vi "Voltage - MeasureAF.vi"() -> ()   [LabVIEW 2017]
doc: "This example demonstrates how to continuously acquire buffered voltage measurements using a DAQmx device.\n\nFor instructions on how to connect your signals to the DAQ device, refer to your device documentation."
uses:
  <vilib>/Utility/error.llb/DialogType.ctl
  <vilib>/DAQmx/read.llb/DAQmx Read (Analog 1D Wfm NChan NSamp).vi
  <vilib>/DAQmx/write.llb/DAQmx Write (Analog 1D Wfm NChan NSamp).vi
  <vilib>/DAQmx/create/channels.llb/DAQmx Create Channel (AO-Voltage-Basic).vi
  <vilib>/DAQmx/configure/timing.llb/DAQmx Timing (Sample Clock).vi
  <vilib>/DAQmx/miscellaneous.llb/DAQmx Fill In Error Info.vi
  <vilib>/DAQmx/create/channels.llb/DAQmx Create Channel (AI-Voltage-Basic).vi
  <vilib>/DAQmx/configure/task.llb/DAQmx Configure Logging (TDMS).vi
  <vilib>/measure/matone.llb/Harmonic Distortion Analyzer N Chan.vi
  <vilib>/measure/matone.llb/Extract Single Tone Information N Chan.vi
  <vilib>/Utility/config.llb/Read Key (Double).vi
  <resource>/objmgr/daqmx.rc
  <vilib>/measure/NI_MAPro.lvlib
  <vilib>/Utility/config.llb/NI_LVConfig.lvlib
  <vilib>/measure/NI_MABase.lvlib
panel:
  out "c7":dbl
  out "c6":dbl
  out "c5":dbl
  out "c4":dbl
  out "c3":dbl
  out "c2":dbl
  out "c1":dbl
  out "c0":dbl
  out "Amplitudes":dbl[](array[numeric]) format="%.2p"
  out "Frequency":dbl[](array[numeric]) format="%.2p"
  out "Channel 7":waveform(dbl)(graph)
  out "Channel 6":waveform(dbl)(graph)
  out "Channel 5":waveform(dbl)(graph)
  out "Channel 4":waveform(dbl)(graph)
  out "Channel 3":waveform(dbl)(graph)
  out "Channel 2":waveform(dbl)(graph)
  out "Channel 1":waveform(dbl)(graph)
  out "Channel 0":waveform(dbl)(graph)
  out "FreqOut":dbl
  out "AmpOut":dbl
  in  "s":bool
  out "x = y?":bool
  in  "Number of Samples display":i32=1000
  in  "Stop 2":bool
  out "Actual Sample Rate 2":dbl=1000.0 format="%0.2f"
  out "Waveform Graph 3":waveform(dbl)[](graph)=[{"t0"=timestamp(0 s since 1904-01-01), "dt"=0.001, "Y"=[]}]
  out "THD":dbl[](array[numeric]) format="%.2p"
  out "Number Sample for avarage AF":i32
  out "stopAI":bool
  out "Time Stop App (s)":i32
  in  "Stop":bool
  out "Waveform Graph":waveform(dbl)[](graph)
  out "Actual Sample Rate":dbl=1000.0 format="%0.2f"
  # "Acquired Data"
  # "Channel0"
  # "Channel1"
  # "Channel2"
  # "Channel3"
  # "Channel4"
  # "Channel5"
  # "Channel6"
  # "Channel7"
  # "Timing Settings"
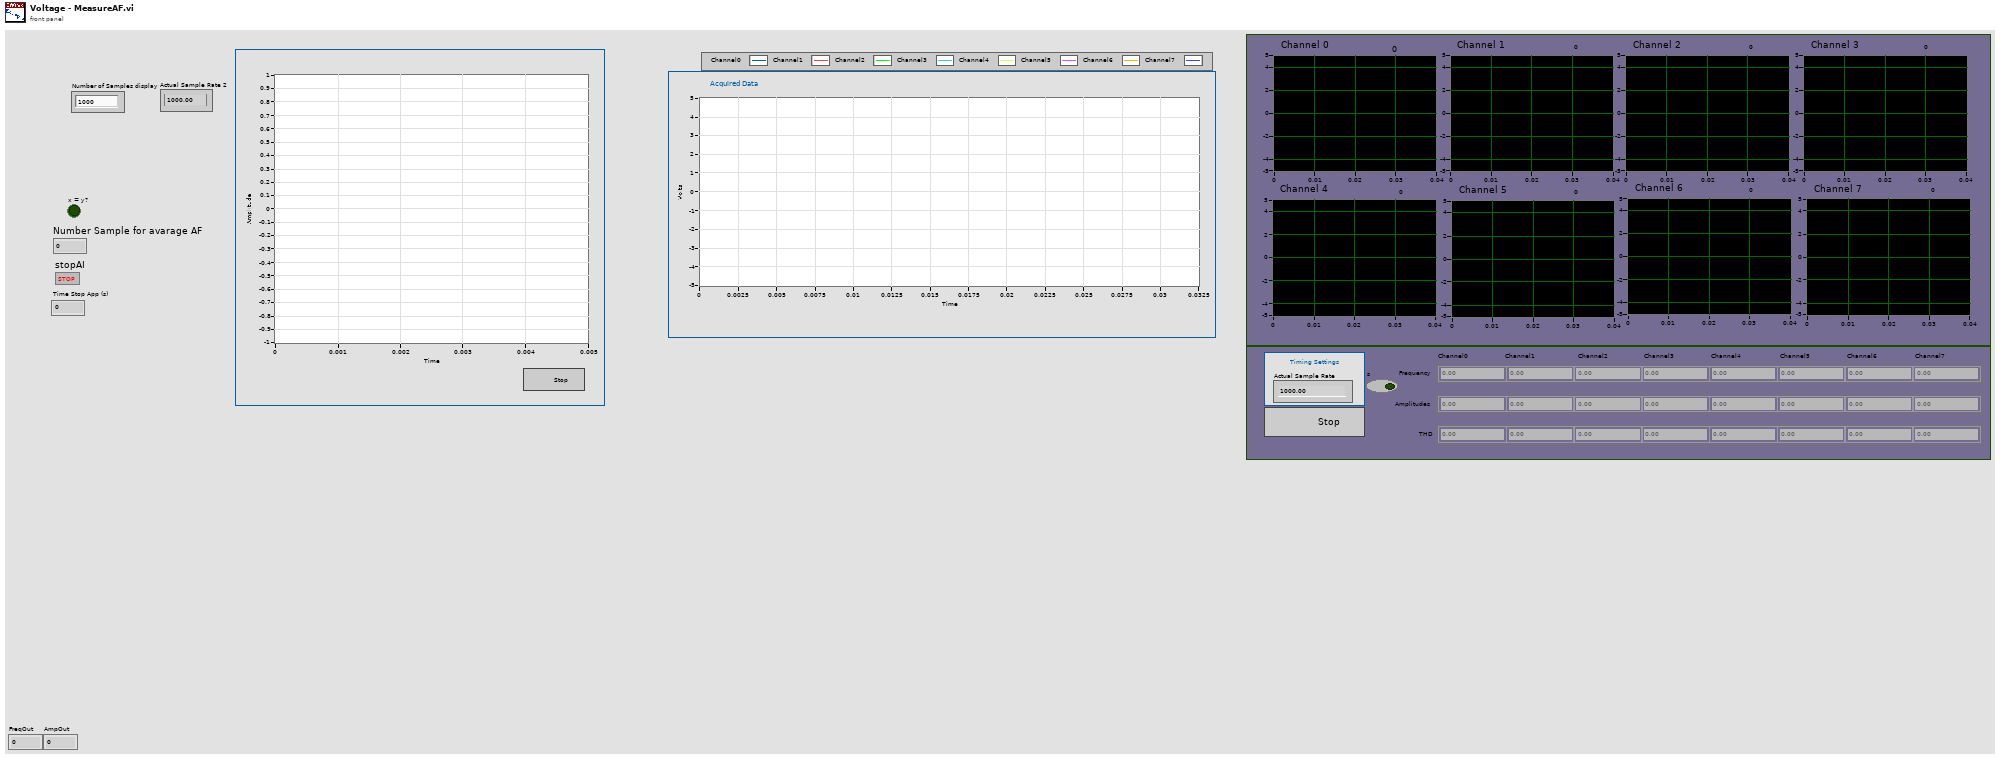
[diagram p1: front panel]
types:
  T1 = typedef "DialogType.ctl" = u16
  T2 = typedef "NI_LVConfig.lvlib/Config Data RefNum.ctl" = refnum<k1>
  T3 = cluster{"Waveform Type":u16, "Amplitude":dbl, "Frequency":dbl}[]
  T4 = cluster{"Waveform Type":u16, "Amplitude":dbl, "Frequency":dbl}
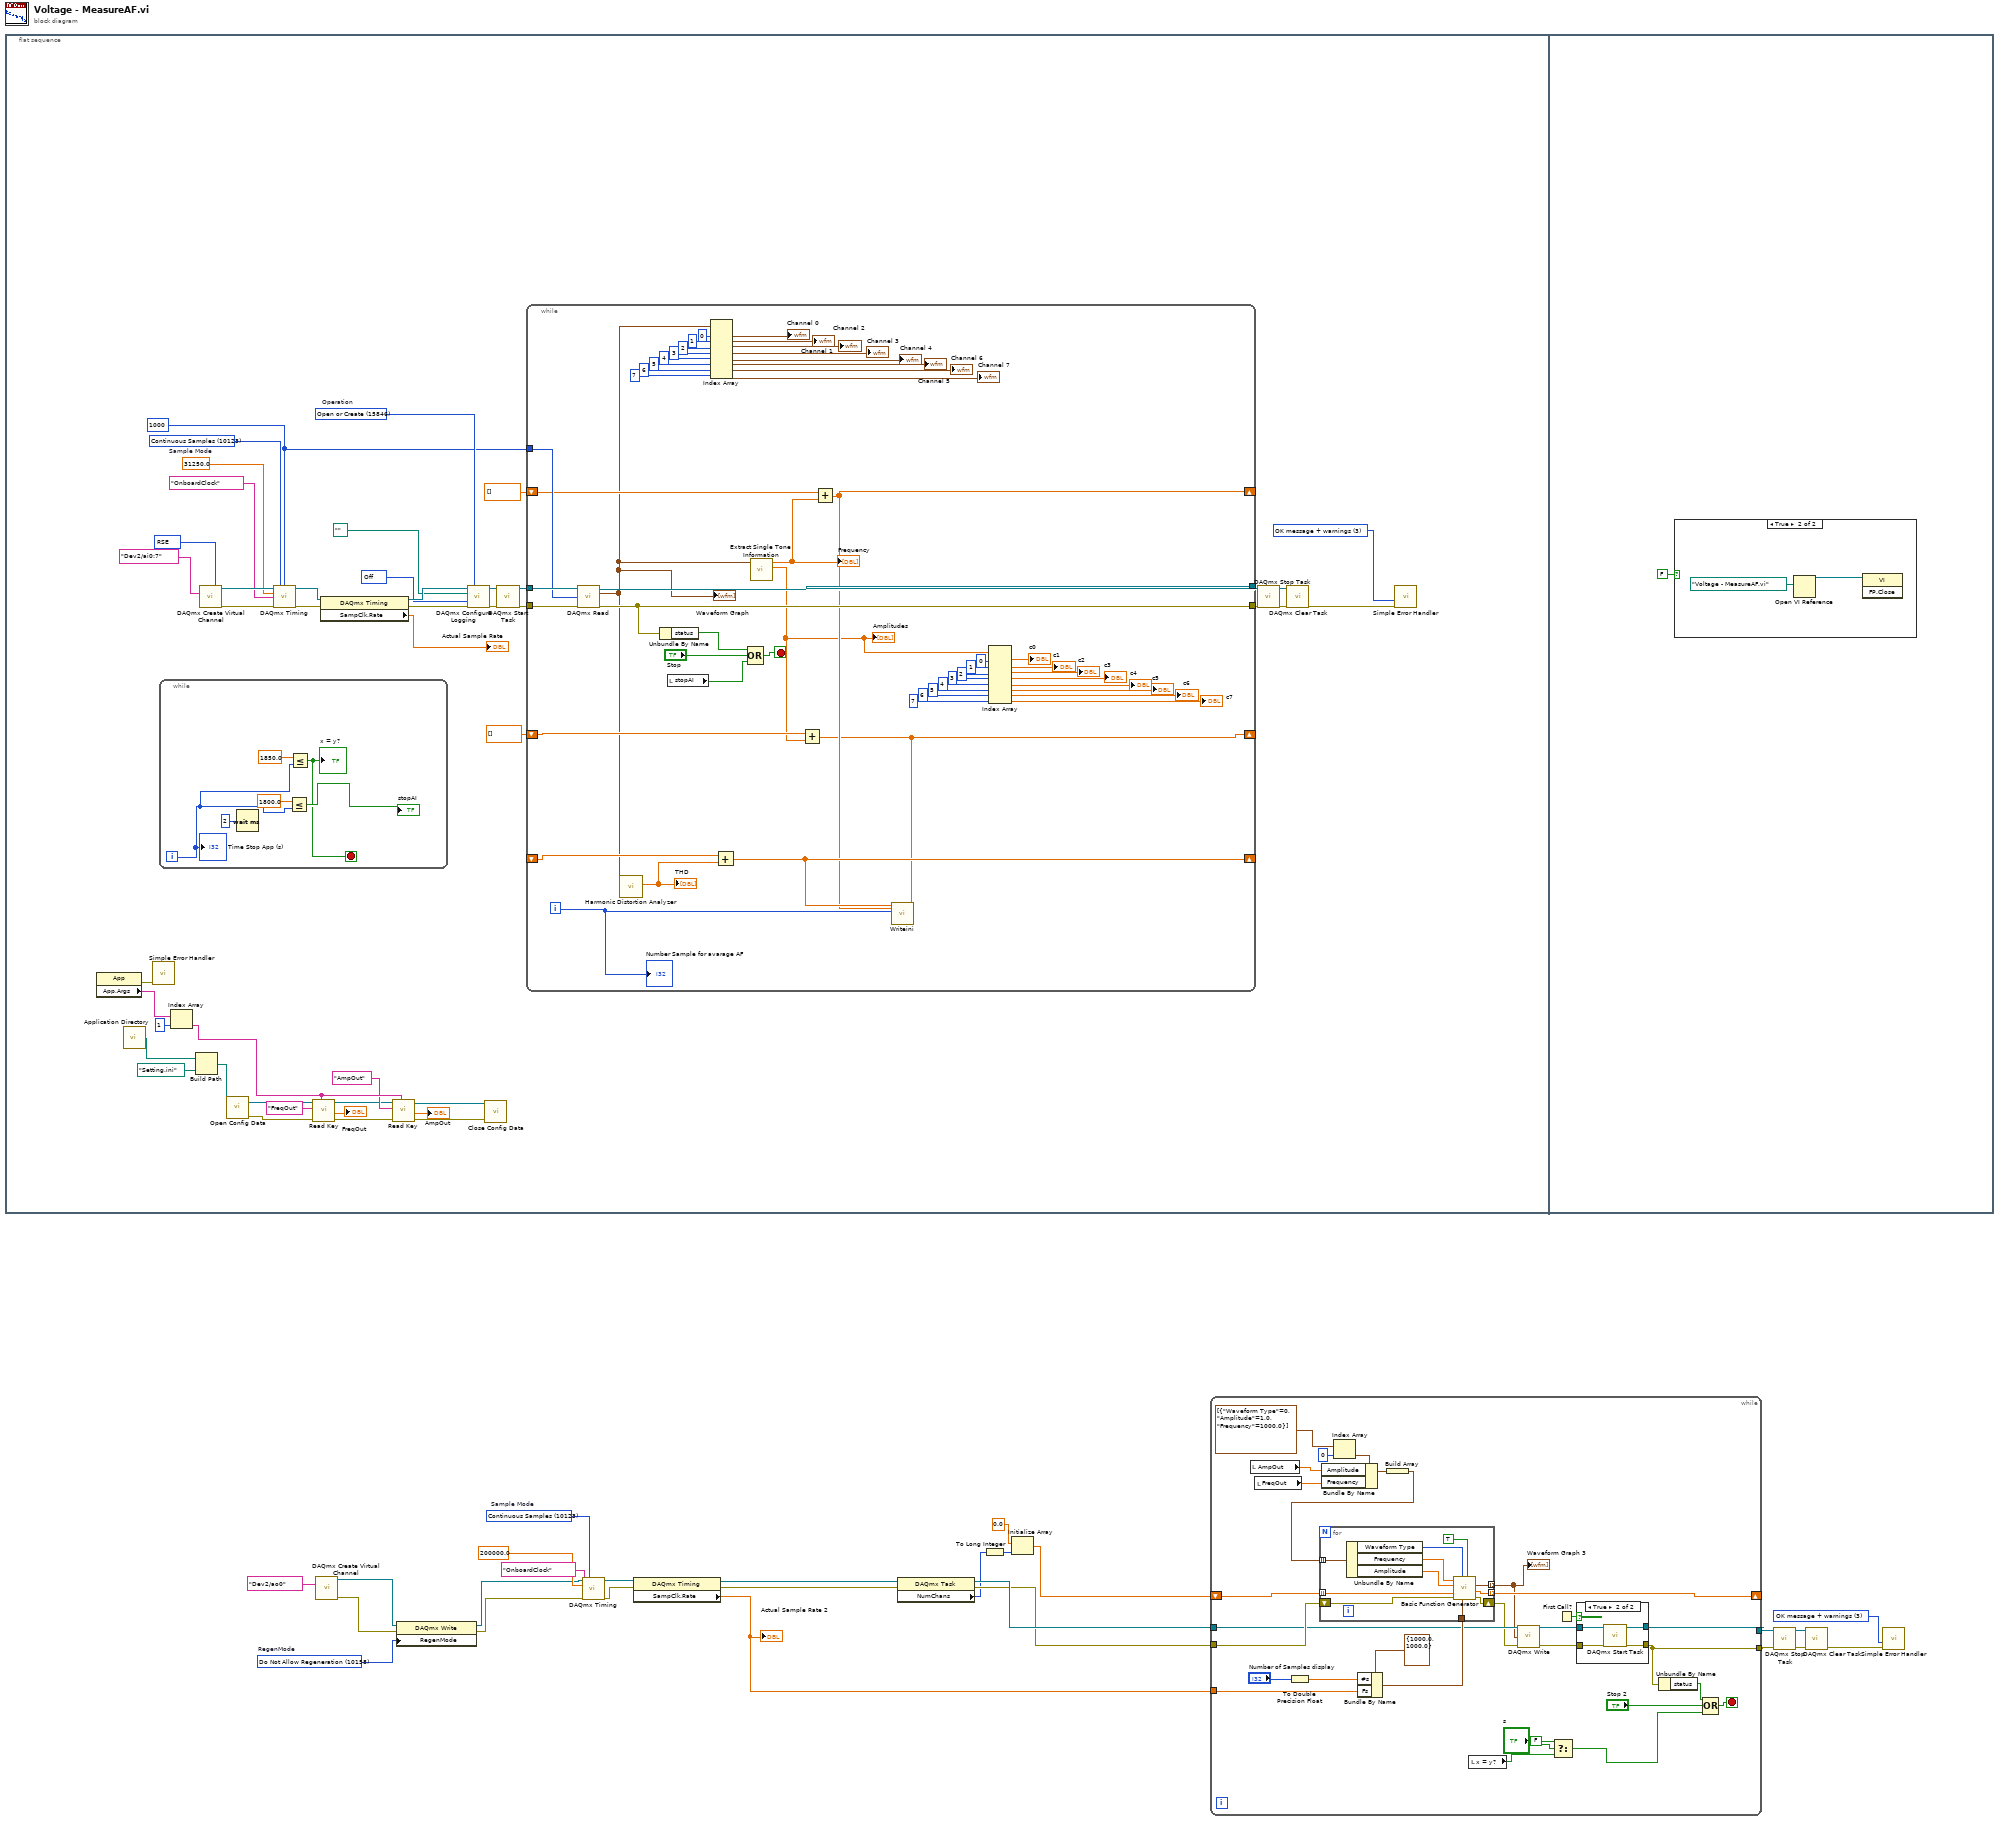
[diagram p0: block diagram]
diagram:
  w5 = 10158 items=["Allow Regeneration"=10097, "Do Not Allow Regeneration"=10158]  # RegenMode
  w15 = T1 3 items=["no dialog", "OK message", "continue or stop message", "OK message + warnings", "continue/stop + warnings"] ("type of dialog (OK msg:1)")
  w24 = 10123 items=["Finite Samples"=10178, "Continuous Samples"=10123, "Hardware Timed Single Point"=12522]  # Sample Mode
  n1 = flat-sequence {
    frame #0 {
      w58 = 1000 ("Number of Samples")
      w48 = 10231 items=["Off"=10231, "Log"=15844, "Log and Read"=15842] ("logging mode")
      w50 = 10083 items=["default"=-1, "RSE"=10083, "NRSE"=10078, "Differential"=10106, "Pseudodifferential"=12529] ("Terminal Configuration")
      w53 = T1 3 items=["no dialog", "OK message", "continue or stop message", "OK message + warnings", "continue/stop + warnings"] ("type of dialog (OK msg:1)")
      w64 = 15846 items=["Open"=10437, "Open or Create"=15846, "Create or Replace"=15847, "Create"=15848]  # Operation
      w69 = 10123 items=["Finite Samples"=10178, "Continuous Samples"=10123, "Hardware Timed Single Point"=12522]  # Sample Mode
      n2 = property class="App"() -> (error out=w34:errorcluster, "App.Args"=w33:string[])  [unwired: 2 in, 1 out]
      n3 = call <vilib>:"Application Directory.vi"() -> ("Application Directory"=w30:path)
      n4 = call <vilib>:"Simple Error Handler.vi"("error in (no error)"=w34) -> ()  [unwired: 1 in, 8 out]
      n5 = while {
        i -> [w74]
        stop <- w72 stop-if-true
        n6 = Wait (ms)(milliseconds to wait=u32 2) -> ()  [unwired: 1 out]
        n7 = Less Or Equal?(x=1800.0, y=w74) -> (x <= y?=→"stopAI":bool)
        n8 = Less Or Equal?(x=1850.0, y=w74) -> (x <= y?=w72:bool)
        "x = y?" <- w72
        "Time Stop App (s)" <- w74
      }
      n9 = Index Array(array=w33, index=1) -> (element=w43:string)
      n10 = Build Path(base path=w30, name or relative path=path "Setting.ini") -> (appended path=w29:path)
      n11 = call-poly <vilib>:"DAQmx Create Virtual Channel.vi"("input terminal configuration"=w50, "physical channels"=tag "Dev2/ai0:7" ("physical Right")) -> ("task out"=w67:refnum<k21>, "error out"=w68:errorcluster)  [unwired: 12 in]
      n12 = call <vilib>:"Open Config Data.vi"("configuration file path"=w29) -> ("error out"=w39:errorcluster, "refnum"=w36:T2)  [unwired: 8 in, 1 out]
      n13 = call-poly <vilib>:"DAQmx Timing.vi"("task/channels in"=w67, "sample mode"=w69, "samples per channel"=w58, "rate"=31250.0 ("Sample Rate"), "source"=tag "OnboardClock", "error in"=w68) -> ("task out"=w71:refnum<k21>, "error out"=w70:errorcluster)  [unwired: 8 in]
      n14 = call-poly <vilib>:"Read Key.vi"("section"=w43, "error in (no error)"=w39, "key"="FreqOut", "refnum"=w36) -> ("error out"=w38:errorcluster, "value"=→"FreqOut":dbl, "refnum out"=w35:T2)  [unwired: 4 in, 1 out]
      n15 = property class="DAQmx Timing"(reference=w71, error in=w70) -> (reference out=w66:refnum<k21>, error out=w65:errorcluster, "SampClk.Rate"=→"Actual Sample Rate":dbl)
      n16 = call-poly <vilib>:"Read Key.vi"("section"=w43, "error in (no error)"=w38, "key"="AmpOut", "refnum"=w35) -> ("error out"=w45:errorcluster, "value"=→"AmpOut":dbl, "refnum out"=w44:T2)  [unwired: 4 in, 1 out]
      n17 = call-poly <vilib>:"DAQmx Configure Logging.vi"("task/channels in"=w66, "operation"=w64, "file path"=path "", "logging mode"=w48, "error in"=w65) -> ("task out"=w52:refnum<k21>, "error out"=w51:errorcluster)  [unwired: 9 in]
      n18 = call <vilib>:"Close Config Data.vi"("error in (no error)"=w45, "refnum"=w44) -> ()  [unwired: 8 in, 2 out]
      n19 = call <vilib>:"DAQmx Start Task.vi"("task/channels in"=w52, "error in"=w51) -> ("task out"=w63:refnum<k21>, "error out"=w62:errorcluster)  [unwired: 12 in]
      n20 = while {
        tunnel: w63 -> [w129]
        tunnel: w62 -> [w128]
        tunnel: [w127] -> w57
        tunnel: [w125] -> w56
        tunnel: w58 -> [w122]
        shift-right: [w114] -> _
        shift-left: dbl[] [] -> [w119]
        shift-right: [w78] -> _
        shift-left: dbl[] [] -> [w118]
        shift-right: [w115] -> _
        shift-left: _ -> [w116]
        i -> [w120]
        stop <- w123 stop-if-true
        n21 = call-poly <vilib>:"DAQmx Read.vi"("task/channels in"=w129, "number of samples per channel"=w122, "error in"=w128) -> ("task out"=w127:refnum<k21>, "data"=w113:waveform(dbl)[], "error out"=w125:errorcluster)  [unwired: 10 in]
        "Waveform Graph" <- w113
        n22 = call-poly <vilib>:"Harmonic Distortion Analyzer.vi"("signals in"=w113) -> ("THD"=w117:dbl[])  [unwired: 5 in, 5 out]
        "THD" <- w117
        n23 = Unbundle By Name(w125) -> ("status"=w124:bool)
        n24 = local read "stopAI"() -> (w121:bool)
        n25 = Index Array(array=w113, index #1=0 ("index"), index #2=1 ("index"), index #3=2 ("index"), index #4=3 ("index"), index #5=4 ("index"), index #6=5 ("index"), index #7=6 ("index"), index #8=7 ("index")) -> (element #1=→"Channel 0":waveform(dbl), element #2=→"Channel 1":waveform(dbl), element #3=→"Channel 2":waveform(dbl), element #4=→"Channel 3":waveform(dbl), element #5=→"Channel 4":waveform(dbl), element #6=→"Channel 5":waveform(dbl), element #7=→"Channel 6":waveform(dbl), element #8=→"Channel 7":waveform(dbl))
        n26 = Add(x=w116, y=w117) -> (x+y=w115:dbl[])
        n27 = Compound Arithmetic op=OR(w124, "Stop", w121) -> (w123:bool)
        n28 = call-poly <vilib>:"Extract Single Tone Information.vi"("time signals in"=w113) -> ("detected amplitudes"=w87:dbl[], "detected frequencies"=w110:dbl[])  [unwired: 5 in, 4 out]
        "Frequency" <- w110
        "Amplitudes" <- w87
        n29 = Add(x=w118, y=w87) -> (x+y=w78:dbl[])
        n30 = Add(x=w119, y=w110) -> (x+y=w114:dbl[])
        n31 = call "Writeini.vi"("Amplitudes"=w78, "Frequency"=w114, "Number Sample for avarage AF"=w120, "THD"=w115) -> ()  [unwired: 8 in]
        n32 = Index Array(array=w87, index #1=0 ("index"), index #2=1 ("index"), index #3=2 ("index"), index #4=3 ("index"), index #5=4 ("index"), index #6=5 ("index"), index #7=6 ("index"), index #8=7 ("index")) -> (element #1=→"c0":dbl, element #2=→"c1":dbl, element #3=→"c2":dbl, element #4=→"c3":dbl, element #5=→"c4":dbl, element #6=→"c5":dbl, element #7=→"c6":dbl, element #8=→"c7":dbl)
        "Number Sample for avarage AF" <- w120
      }
      n33 = call <vilib>:"DAQmx Stop Task.vi"("task/channels in"=w57, "error in"=w56) -> ("task out"=w54:refnum<k21>, "error out"=w55:errorcluster)  [unwired: 12 in]
      n34 = call <vilib>:"DAQmx Clear Task.vi"("task in"=w54, "error in"=w55) -> ("error out"=w61:errorcluster)  [unwired: 13 in]
      n35 = call <vilib>:"Simple Error Handler.vi"("type of dialog (OK msg:1)"=w53, "error in (no error)"=w61) -> ()  [unwired: 3 in, 5 out]
    }
    frame #1 {
      n36 = case shown="True" FALSE {
        frame False {
        }
        frame True {
          n37 = Open VI Reference(vi path=path "Voltage - MeasureAF.vi") -> (vi reference=w131:refnum<vi>)  [unwired: 5 in, 1 out]
          n38 = invoke class="VI" method="FP.Close"(reference=w131) -> ()  [unwired: 2 in, 3 out]
        }
      }
    }
  }
  n39 = call-poly <vilib>:"DAQmx Create Virtual Channel.vi"("physical channels"=tag "Dev2/ao0" ("Physical Channel(s)")) -> ("task out"=w3:refnum<k21>, "error out"=w2:errorcluster)  [unwired: 13 in]
  n40 = property class="DAQmx Write"(reference=w3, error in=w2, "RegenMode"=w5) -> (reference out=w4:refnum<k21>, error out=w1:errorcluster)
  n41 = call-poly <vilib>:"DAQmx Timing.vi"("task/channels in"=w4, "sample mode"=w24, "rate"=200000.0 ("Sample Rate"), "source"=tag "OnboardClock", "error in"=w1) -> ("task out"=w26:refnum<k21>, "error out"=w25:errorcluster)  [unwired: 9 in]
  n42 = property class="DAQmx Timing"(reference=w26, error in=w25) -> (reference out=w10:refnum<k21>, error out=w9:errorcluster, "SampClk.Rate"=w20:dbl)
  "Actual Sample Rate 2" <- w20
  n43 = property class="DAQmx Task"(reference=w10, error in=w9) -> (reference out=w12:refnum<k21>, error out=w11:errorcluster, "NumChans"=w8:u32)
  n44 = To Long Integer(number=w8) -> (32bit integer=w7:i32)
  n45 = Initialize Array(0.0 ("element"), w7) -> (w13:dbl[])
  n46 = while {
    tunnel: w11 -> [w162]
    tunnel: w20 -> [w160]
    tunnel: w12 -> [w158]
    tunnel: [w151] -> w17
    tunnel: [w150] -> w16
    shift-right: [w146] -> _
    shift-left: w13 -> [w145]
    stop <- w148 stop-if-true
    n47 = local read "AmpOut"() -> (w133:dbl)
    n48 = local read "FreqOut"() -> (w134:dbl)
    n49 = To Double Precision Float(number="Number of Samples display") -> (double precision float=w154:dbl)
    n50 = Index Array(array=T3 [{"Waveform Type"=0, "Amplitude"=1.0, "Frequency"=1000.0}] ("Output Array"), index=0) -> (element=w138:T4)
    n51 = Bundle By Name(cluster=w138, "Amplitude"=w133, "Frequency"=w134) -> (w139:T4)
    n52 = Bundle By Name(cluster=cluster{"Fs":dbl, "#s":dbl} {"Fs"=1000.0, "#s"=1000.0} ("sampling info"), "#s"=w154, "Fs"=w160) -> (w159:cluster{"Fs":dbl, "#s":dbl})
    n53 = Build Array(w139) -> (w135:T3)
    n54 = for {
      tunnel: w159 -> [w178]
      tunnel: w135 -> [w176] mode=indexing
      tunnel: [w172] -> w144 mode=indexing
      tunnel: [w171] -> w146 mode=indexing
      tunnel: w145 -> [w169] mode=indexing
      shift-right: [w177] -> w155
      shift-left: w162 -> [w179]
      n55 = Unbundle By Name(w176) -> ("Waveform Type"=w175:u16, "Frequency"=w174:dbl, "Amplitude"=w173:dbl)
      n56 = call <vilib>:"Basic Function Generator.vi"("reset signal"=TRUE, "sampling info"=w178, "signal type"=w175, "error in (no error)"=w179, "phase"=w169, "amplitude"=w173, "frequency"=w174) -> ("error out"=w177:errorcluster, "phase out"=w171:dbl, "signal out"=w172:waveform(dbl))  [unwired: 2 in]
    }
    "Waveform Graph 3" <- w144
    n57 = local read "x = y?"() -> (w142:bool)
    n58 = call-poly <vilib>:"DAQmx Write.vi"("task/channels in"=w158, "data"=w144, "error in"=w155) -> ("task out"=w157:refnum<k21>, "error out"=w156:errorcluster)  [unwired: 10 in, 1 out]
    n59 = Select(t=FALSE, s="s", f=w142) -> (s? t:f=w143:bool)
    n60 = First Call?() -> (First Call?: T/F=w152:bool)
    n61 = case shown="True" w152 {
      tunnel: w157 -> [w163 w168]
      tunnel: w156 -> [w164 w167]
      tunnel: [w163 w166] -> w151
      tunnel: [w164 w165] -> w150
      frame False {
      }
      frame True {
        n62 = call <vilib>:"DAQmx Start Task.vi"("task/channels in"=w168, "error in"=w167) -> ("task out"=w166:refnum<k21>, "error out"=w165:errorcluster)  [unwired: 12 in]
      }
    }
    n63 = Unbundle By Name(w150) -> ("status"=w147:bool)
    n64 = Compound Arithmetic op=OR(w147, "Stop 2", w143) -> (w148:bool)
  }
  n65 = call <vilib>:"DAQmx Stop Task.vi"("task/channels in"=w17, "error in"=w16) -> ("task out"=w19:refnum<k21>, "error out"=w18:errorcluster)  [unwired: 12 in]
  n66 = call <vilib>:"DAQmx Clear Task.vi"("task in"=w19, "error in"=w18) -> ("error out"=w23:errorcluster)  [unwired: 13 in]
  n67 = call <vilib>:"Simple Error Handler.vi"("type of dialog (OK msg:1)"=w15, "error in (no error)"=w23) -> ()  [unwired: 3 in, 5 out]
